vi "LlenarTabla.vi"(8 "error in (no error)":errorcluster, 10 "Tabla":T1(ring), 11 "Prueba32 in":refnum<class "Prueba33.lvclass">) -> (0 "error out":errorcluster, 3 "Prueba32 out":refnum<class "Prueba33.lvclass">)   [LabVIEW 2019, in "Prueba33.lvclass"]
uses:
  Prueba33.lvclass
  Prueba33.lvclass/Prueba33.ctl
panel:
  out "Tabla":string[][](table)=[["63"], ["125"], ["250"], ["500"], ["1000"], ["2000"], ["4000"], ["8000"]]
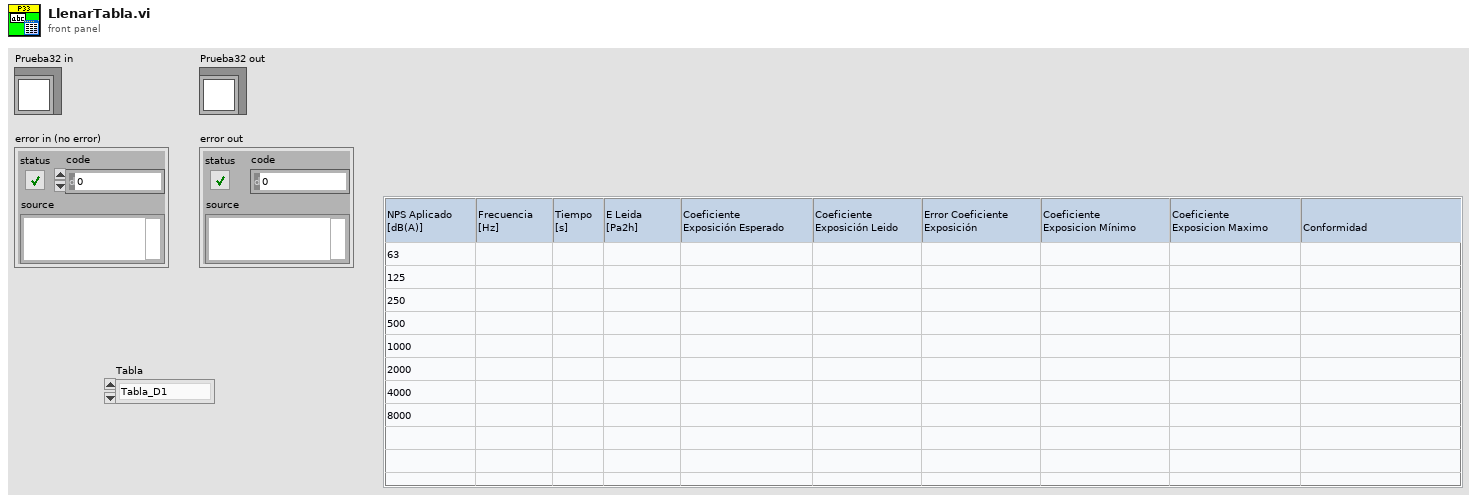
[diagram p1: front panel]
types:
  T1 = enum16{"Tabla_D1", "Tabla_D2", "Tabla_D3", "Tabla_D4"}
  T2 = cluster{"ControlName":string, "ControlReference":refnum<vi>}[]
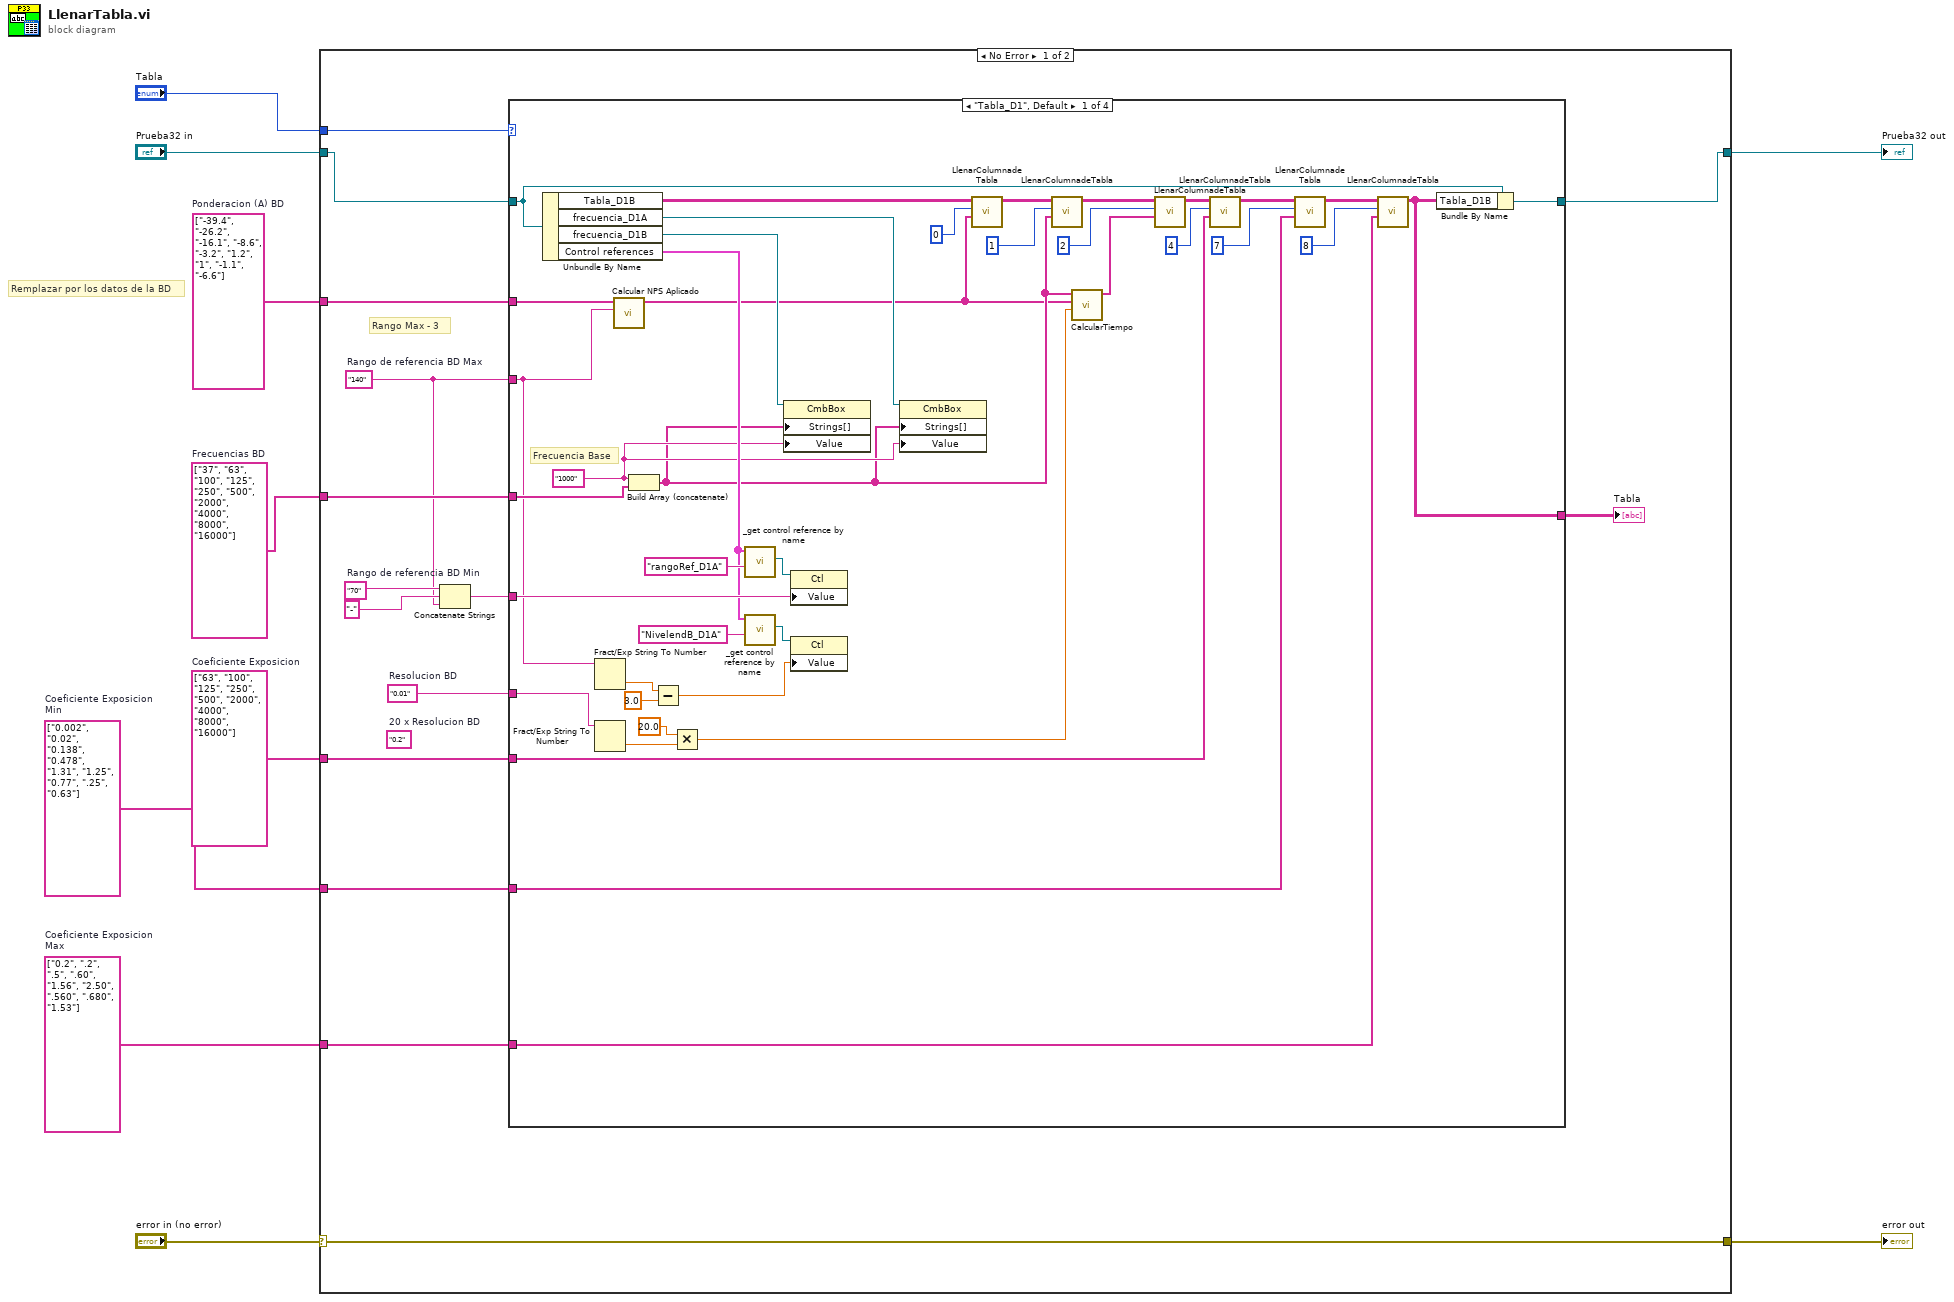
[diagram p0: block diagram]
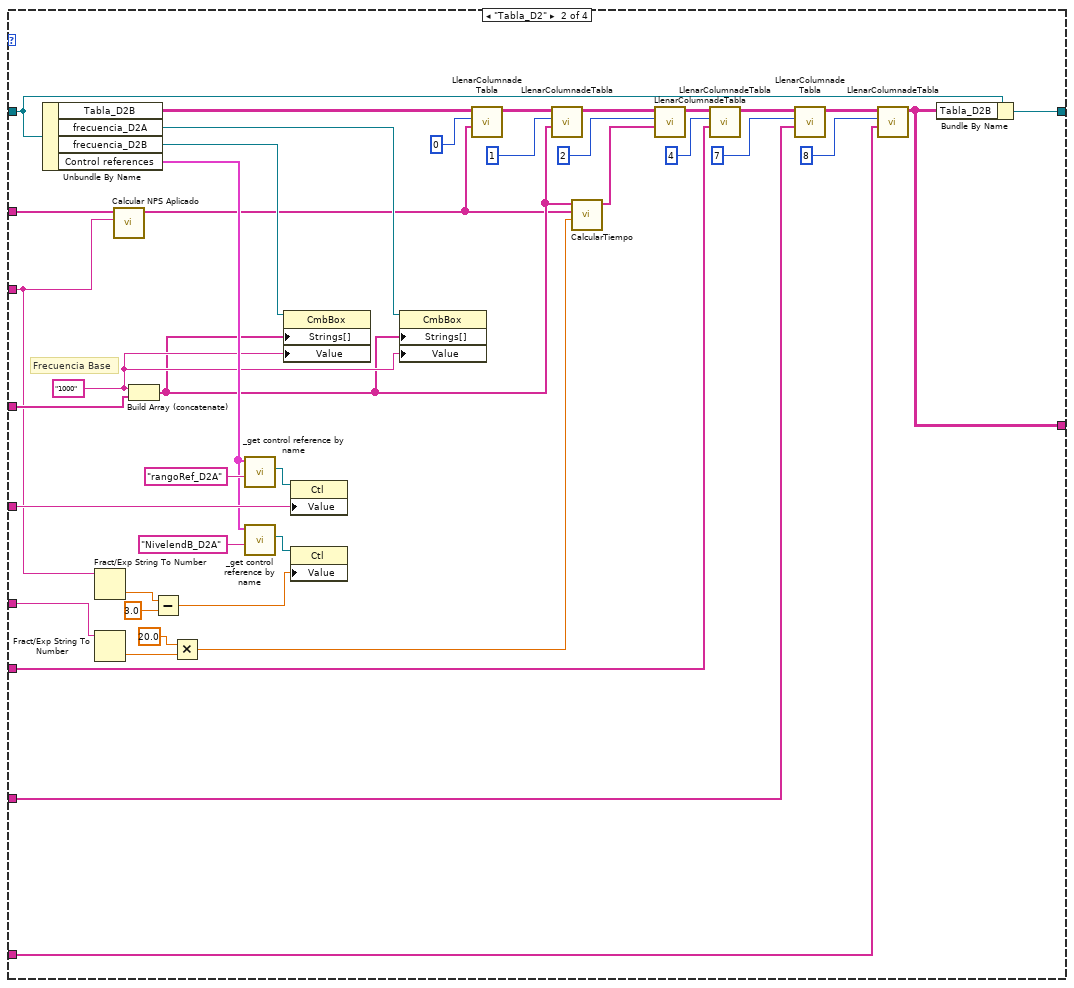
[diagram p2: hidden frame]
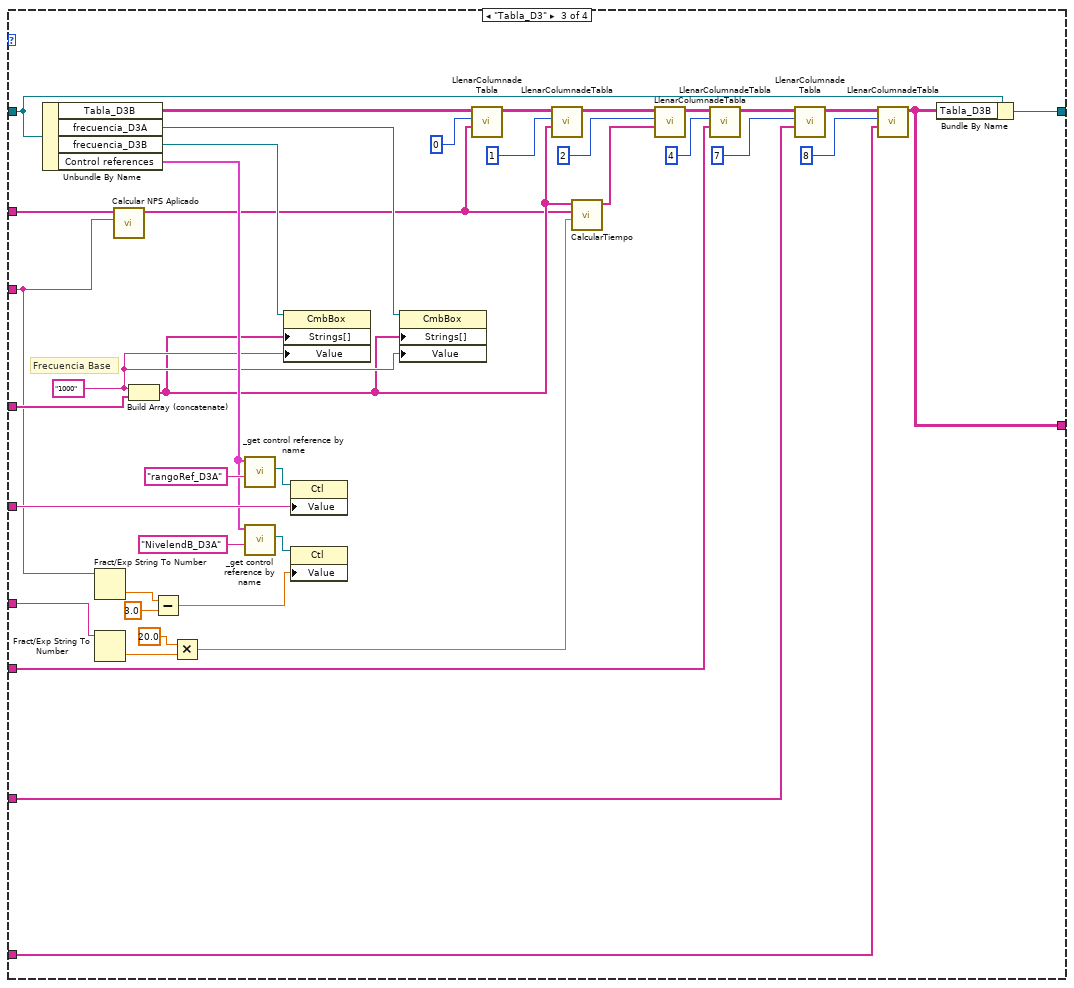
[diagram p3: hidden frame]
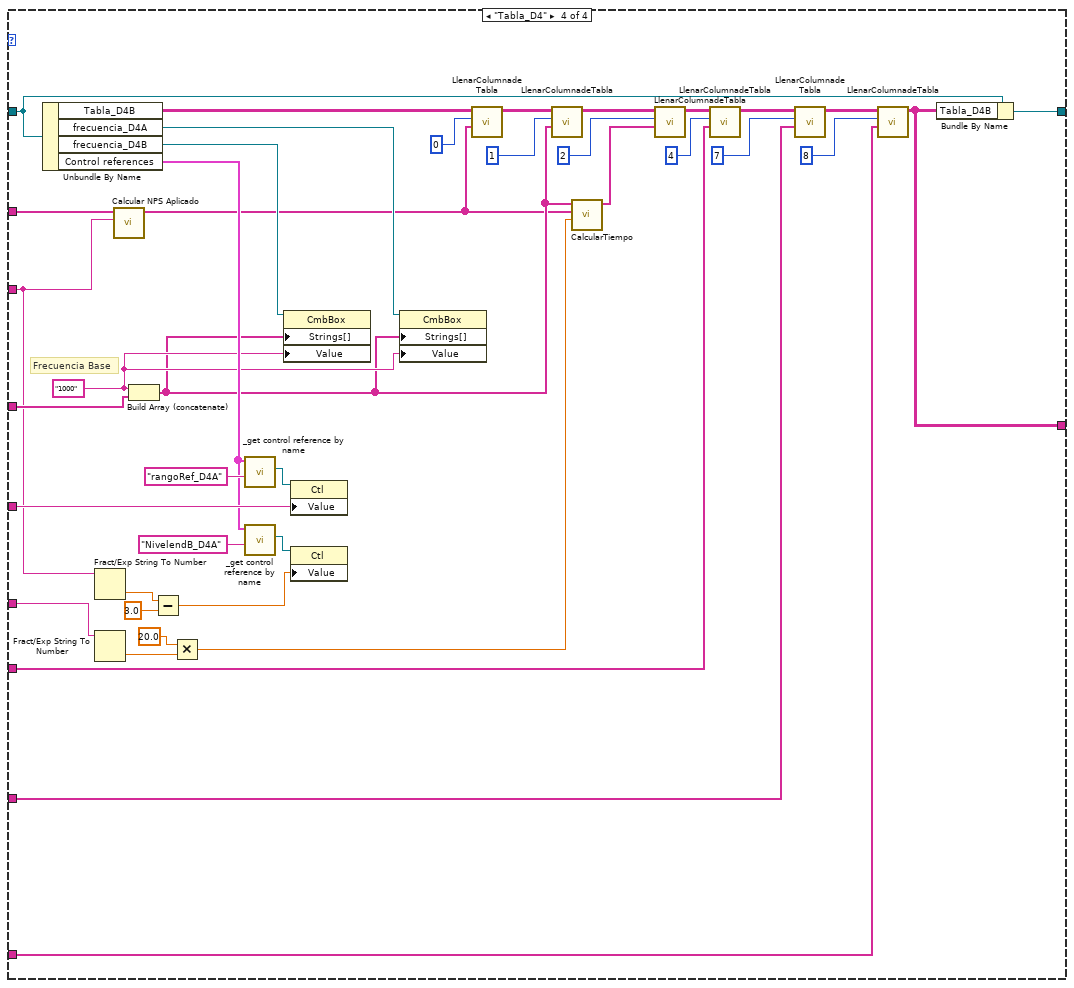
[diagram p4: hidden frame]
diagram:
  w1 = string[] ["0.2", ".2", ".5", ".60", "1.56", "2.50", ".560", ".680", "1.53"]  # Coeficiente Exposicion Max
  w2 = string[] ["0.002", "0.02", "0.138", "0.478", "1.31", "1.25", "0.77", ".25", "0.63"]  # Coeficiente Exposicion Min
  w3 = string[] ["63", "100", "125", "250", "500", "2000", "4000", "8000", "16000"]  # Coeficiente Exposicion
  w4 = string[] ["37", "63", "100", "125", "250", "500", "2000", "4000", "8000", "16000"]  # Frecuencias BD
  w5 = string[] ["-39.4", "-26.2", "-16.1", "-8.6", "-3.2", "1.2", "1", "-1.1", "-6.6"]  # Ponderacion (A) BD
  # "Remplazar por los datos de la BD"
  n1 = case shown="No Error" "error in (no error)" {
    selector: "error in (no error)" -> [w25 w186]
    tunnel: [w25 w186] -> w8
    tunnel: [w24 w187] -> w9
    tunnel: "Prueba32 in" -> [w23 w187]
    tunnel: "Tabla" -> [w22 _]
    tunnel: w5 -> [w21 _]
    tunnel: w4 -> [w20 _]
    tunnel: w3 -> [w19 _]
    tunnel: w2 -> [w18 _]
    tunnel: w1 -> [w17 _]
    frame No Error {
      w11 = "0.01"  # Resolucion BD
      (unwired) "0.2"  # 20 x Resolucion BD
      w12 = "140"  # Rango de referencia BD Max
      w15 = "70"  # Rango de referencia BD Min
      # "Rango Max - 3"
      n2 = Concatenate Strings(w15, "-", w12) -> (w13:string)
      n3 = case shown="\"Tabla_D1\", Default" w22 {
        tunnel: [w64 w104 w144 w184] -> w24
        tunnel: w23 -> [w63 w103 w143 w183]
        tunnel: w12 -> [w40 w80 w120 w160]
        tunnel: w21 -> [w61 w101 w141 w181]
        tunnel: w20 -> [w58 w98 w138 w178]
        tunnel: w19 -> [w54 w94 w134 w174]
        tunnel: w18 -> [w48 w88 w128 w168]
        tunnel: w17 -> [w47 w87 w127 w167]
        tunnel: [w46 w86 w126 w166] -> w16
        tunnel: w13 -> [w43 w83 w123 w163]
        tunnel: w11 -> [w30 w70 w110 w150]
        frame "Tabla_D1", Default {
          w33 = "1000"
          # "Frecuencia Base"
          n4 = Unbundle By Name(w63) -> ("Tabla_D1B"=w65:string[][], "frecuencia_D1A"=w34:refnum<vi>, "frecuencia_D1B"=w35:refnum<vi>, "Control references"=w36:T2)
          n5 = Fract/Exp String To Number(string=w40) -> (number=w39:dbl)  [unwired: 3 in, 1 out]
          n6 = Fract/Exp String To Number(string=w30) -> (number=w29:dbl)  [unwired: 3 in, 1 out]
          n7 = call "Calcular NPS Aplicado.vi"("Rango de MAX de referencia BD"=w40, "Ponderacion BD"=w61) -> ("NPS Aplicado"=w31:string[])  [unwired: 9 in]
          n8 = Build Array (concatenate)(w33, w58) -> (w32:string[])
          n9 = Subtract(x=w39, y=3.0) -> (x-y=w37:dbl)
          n10 = Multiply(x=20.0, y=w29) -> (x*y=w27:dbl)
          n11 = call "_get control reference by name.vi"("Control name"="rangoRef_D1A", "Control references"=w36) -> ("Ctl Refnum"=w44:refnum<vi>)  [unwired: 4 in, 1 out]
          n12 = call "_get control reference by name.vi"("Control name"="NivelendB_D1A", "Control references"=w36) -> ("Ctl Refnum"=w41:refnum<vi>)  [unwired: 4 in, 1 out]
          n13 = property class="CmbBox"(reference=w35, "Strings[]"=w32, "Value"=w33) -> ()  [unwired: 1 in, 2 out]
          n14 = property class="Ctl"(reference=w44, "Value"=w43) -> ()  [unwired: 1 in, 2 out]
          n15 = property class="Ctl"(reference=w41, "Value"=w37) -> ()  [unwired: 1 in, 2 out]
          n16 = property class="CmbBox"(reference=w34, "Strings[]"=w32, "Value"=w33) -> ()  [unwired: 1 in, 2 out]
          n17 = call "LlenarColumnadeTabla.vi"("Data"=w31, "Col. Number"=0, "Tabla in"=w65) -> ("Tabla out"=w59:string[][])  [unwired: 8 in]
          n18 = call "LlenarColumnadeTabla.vi"("Data"=w32, "Col. Number"=1, "Tabla in"=w59) -> ("Tabla out"=w57:string[][])  [unwired: 8 in]
          n19 = call "CalcularTiempo.vi"("20xResolucion"=w27, "NPS Aplicado"=w31, "Frecuencias"=w32) -> ("Tiempo"=w26:string[])  [unwired: 8 in]
          n20 = call "LlenarColumnadeTabla.vi"("Data"=w26, "Col. Number"=2, "Tabla in"=w57) -> ("Tabla out"=w55:string[][])  [unwired: 8 in]
          n21 = call "LlenarColumnadeTabla.vi"("Data"=w54, "Col. Number"=4, "Tabla in"=w55) -> ("Tabla out"=w52:string[][])  [unwired: 8 in]
          n22 = call "LlenarColumnadeTabla.vi"("Data"=w48, "Col. Number"=7, "Tabla in"=w52) -> ("Tabla out"=w51:string[][])  [unwired: 8 in]
          n23 = call "LlenarColumnadeTabla.vi"("Data"=w47, "Col. Number"=8, "Tabla in"=w51) -> ("Tabla out"=w46:string[][])  [unwired: 8 in]
          n24 = Bundle By Name(cluster=w63, "Tabla_D1B"=w46) -> (w64:refnum<class "Prueba33.lvclass">)
        }
        frame "Tabla_D2" {
          w73 = "1000"
          # "Frecuencia Base"
          n25 = Unbundle By Name(w103) -> ("Tabla_D2B"=w105:string[][], "frecuencia_D2A"=w74:refnum<vi>, "frecuencia_D2B"=w75:refnum<vi>, "Control references"=w76:T2)
          n26 = Fract/Exp String To Number(string=w80) -> (number=w79:dbl)  [unwired: 3 in, 1 out]
          n27 = Fract/Exp String To Number(string=w70) -> (number=w69:dbl)  [unwired: 3 in, 1 out]
          n28 = call "Calcular NPS Aplicado.vi"("Rango de MAX de referencia BD"=w80, "Ponderacion BD"=w101) -> ("NPS Aplicado"=w71:string[])  [unwired: 9 in]
          n29 = Build Array (concatenate)(w73, w98) -> (w72:string[])
          n30 = Subtract(x=w79, y=3.0) -> (x-y=w77:dbl)
          n31 = Multiply(x=20.0, y=w69) -> (x*y=w67:dbl)
          n32 = call "_get control reference by name.vi"("Control name"="rangoRef_D2A", "Control references"=w76) -> ("Ctl Refnum"=w84:refnum<vi>)  [unwired: 4 in, 1 out]
          n33 = call "_get control reference by name.vi"("Control name"="NivelendB_D2A", "Control references"=w76) -> ("Ctl Refnum"=w81:refnum<vi>)  [unwired: 4 in, 1 out]
          n34 = property class="CmbBox"(reference=w75, "Strings[]"=w72, "Value"=w73) -> ()  [unwired: 1 in, 2 out]
          n35 = property class="Ctl"(reference=w84, "Value"=w83) -> ()  [unwired: 1 in, 2 out]
          n36 = property class="Ctl"(reference=w81, "Value"=w77) -> ()  [unwired: 1 in, 2 out]
          n37 = property class="CmbBox"(reference=w74, "Strings[]"=w72, "Value"=w73) -> ()  [unwired: 1 in, 2 out]
          n38 = call "LlenarColumnadeTabla.vi"("Data"=w71, "Col. Number"=0, "Tabla in"=w105) -> ("Tabla out"=w99:string[][])  [unwired: 8 in]
          n39 = call "LlenarColumnadeTabla.vi"("Data"=w72, "Col. Number"=1, "Tabla in"=w99) -> ("Tabla out"=w97:string[][])  [unwired: 8 in]
          n40 = call "CalcularTiempo.vi"("20xResolucion"=w67, "NPS Aplicado"=w71, "Frecuencias"=w72) -> ("Tiempo"=w66:string[])  [unwired: 8 in]
          n41 = call "LlenarColumnadeTabla.vi"("Data"=w66, "Col. Number"=2, "Tabla in"=w97) -> ("Tabla out"=w95:string[][])  [unwired: 8 in]
          n42 = call "LlenarColumnadeTabla.vi"("Data"=w94, "Col. Number"=4, "Tabla in"=w95) -> ("Tabla out"=w92:string[][])  [unwired: 8 in]
          n43 = call "LlenarColumnadeTabla.vi"("Data"=w88, "Col. Number"=7, "Tabla in"=w92) -> ("Tabla out"=w91:string[][])  [unwired: 8 in]
          n44 = call "LlenarColumnadeTabla.vi"("Data"=w87, "Col. Number"=8, "Tabla in"=w91) -> ("Tabla out"=w86:string[][])  [unwired: 8 in]
          n45 = Bundle By Name(cluster=w103, "Tabla_D2B"=w86) -> (w104:refnum<class "Prueba33.lvclass">)
        }
        frame "Tabla_D3" {
          w113 = "1000"
          # "Frecuencia Base"
          n46 = Unbundle By Name(w143) -> ("Tabla_D3B"=w145:string[][], "frecuencia_D3A"=w114:refnum<vi>, "frecuencia_D3B"=w115:refnum<vi>, "Control references"=w116:T2)
          n47 = Fract/Exp String To Number(string=w120) -> (number=w119:dbl)  [unwired: 3 in, 1 out]
          n48 = Fract/Exp String To Number(string=w110) -> (number=w109:dbl)  [unwired: 3 in, 1 out]
          n49 = call "Calcular NPS Aplicado.vi"("Rango de MAX de referencia BD"=w120, "Ponderacion BD"=w141) -> ("NPS Aplicado"=w111:string[])  [unwired: 9 in]
          n50 = Build Array (concatenate)(w113, w138) -> (w112:string[])
          n51 = Subtract(x=w119, y=3.0) -> (x-y=w117:dbl)
          n52 = Multiply(x=20.0, y=w109) -> (x*y=w107:dbl)
          n53 = call "_get control reference by name.vi"("Control name"="rangoRef_D3A", "Control references"=w116) -> ("Ctl Refnum"=w124:refnum<vi>)  [unwired: 4 in, 1 out]
          n54 = call "_get control reference by name.vi"("Control name"="NivelendB_D3A", "Control references"=w116) -> ("Ctl Refnum"=w121:refnum<vi>)  [unwired: 4 in, 1 out]
          n55 = property class="CmbBox"(reference=w115, "Strings[]"=w112, "Value"=w113) -> ()  [unwired: 1 in, 2 out]
          n56 = property class="Ctl"(reference=w124, "Value"=w123) -> ()  [unwired: 1 in, 2 out]
          n57 = property class="Ctl"(reference=w121, "Value"=w117) -> ()  [unwired: 1 in, 2 out]
          n58 = property class="CmbBox"(reference=w114, "Strings[]"=w112, "Value"=w113) -> ()  [unwired: 1 in, 2 out]
          n59 = call "LlenarColumnadeTabla.vi"("Data"=w111, "Col. Number"=0, "Tabla in"=w145) -> ("Tabla out"=w139:string[][])  [unwired: 8 in]
          n60 = call "LlenarColumnadeTabla.vi"("Data"=w112, "Col. Number"=1, "Tabla in"=w139) -> ("Tabla out"=w137:string[][])  [unwired: 8 in]
          n61 = call "CalcularTiempo.vi"("20xResolucion"=w107, "NPS Aplicado"=w111, "Frecuencias"=w112) -> ("Tiempo"=w106:string[])  [unwired: 8 in]
          n62 = call "LlenarColumnadeTabla.vi"("Data"=w106, "Col. Number"=2, "Tabla in"=w137) -> ("Tabla out"=w135:string[][])  [unwired: 8 in]
          n63 = call "LlenarColumnadeTabla.vi"("Data"=w134, "Col. Number"=4, "Tabla in"=w135) -> ("Tabla out"=w132:string[][])  [unwired: 8 in]
          n64 = call "LlenarColumnadeTabla.vi"("Data"=w128, "Col. Number"=7, "Tabla in"=w132) -> ("Tabla out"=w131:string[][])  [unwired: 8 in]
          n65 = call "LlenarColumnadeTabla.vi"("Data"=w127, "Col. Number"=8, "Tabla in"=w131) -> ("Tabla out"=w126:string[][])  [unwired: 8 in]
          n66 = Bundle By Name(cluster=w143, "Tabla_D3B"=w126) -> (w144:refnum<class "Prueba33.lvclass">)
        }
        frame "Tabla_D4" {
          w153 = "1000"
          # "Frecuencia Base"
          n67 = Unbundle By Name(w183) -> ("Tabla_D4B"=w185:string[][], "frecuencia_D4A"=w154:refnum<vi>, "frecuencia_D4B"=w155:refnum<vi>, "Control references"=w156:T2)
          n68 = Fract/Exp String To Number(string=w160) -> (number=w159:dbl)  [unwired: 3 in, 1 out]
          n69 = Fract/Exp String To Number(string=w150) -> (number=w149:dbl)  [unwired: 3 in, 1 out]
          n70 = call "Calcular NPS Aplicado.vi"("Rango de MAX de referencia BD"=w160, "Ponderacion BD"=w181) -> ("NPS Aplicado"=w151:string[])  [unwired: 9 in]
          n71 = Build Array (concatenate)(w153, w178) -> (w152:string[])
          n72 = Subtract(x=w159, y=3.0) -> (x-y=w157:dbl)
          n73 = Multiply(x=20.0, y=w149) -> (x*y=w147:dbl)
          n74 = call "_get control reference by name.vi"("Control name"="rangoRef_D4A", "Control references"=w156) -> ("Ctl Refnum"=w164:refnum<vi>)  [unwired: 4 in, 1 out]
          n75 = call "_get control reference by name.vi"("Control name"="NivelendB_D4A", "Control references"=w156) -> ("Ctl Refnum"=w161:refnum<vi>)  [unwired: 4 in, 1 out]
          n76 = property class="CmbBox"(reference=w155, "Strings[]"=w152, "Value"=w153) -> ()  [unwired: 1 in, 2 out]
          n77 = property class="Ctl"(reference=w164, "Value"=w163) -> ()  [unwired: 1 in, 2 out]
          n78 = property class="Ctl"(reference=w161, "Value"=w157) -> ()  [unwired: 1 in, 2 out]
          n79 = property class="CmbBox"(reference=w154, "Strings[]"=w152, "Value"=w153) -> ()  [unwired: 1 in, 2 out]
          n80 = call "LlenarColumnadeTabla.vi"("Data"=w151, "Col. Number"=0, "Tabla in"=w185) -> ("Tabla out"=w179:string[][])  [unwired: 8 in]
          n81 = call "LlenarColumnadeTabla.vi"("Data"=w152, "Col. Number"=1, "Tabla in"=w179) -> ("Tabla out"=w177:string[][])  [unwired: 8 in]
          n82 = call "CalcularTiempo.vi"("20xResolucion"=w147, "NPS Aplicado"=w151, "Frecuencias"=w152) -> ("Tiempo"=w146:string[])  [unwired: 8 in]
          n83 = call "LlenarColumnadeTabla.vi"("Data"=w146, "Col. Number"=2, "Tabla in"=w177) -> ("Tabla out"=w175:string[][])  [unwired: 8 in]
          n84 = call "LlenarColumnadeTabla.vi"("Data"=w174, "Col. Number"=4, "Tabla in"=w175) -> ("Tabla out"=w172:string[][])  [unwired: 8 in]
          n85 = call "LlenarColumnadeTabla.vi"("Data"=w168, "Col. Number"=7, "Tabla in"=w172) -> ("Tabla out"=w171:string[][])  [unwired: 8 in]
          n86 = call "LlenarColumnadeTabla.vi"("Data"=w167, "Col. Number"=8, "Tabla in"=w171) -> ("Tabla out"=w166:string[][])  [unwired: 8 in]
          n87 = Bundle By Name(cluster=w183, "Tabla_D4B"=w166) -> (w184:refnum<class "Prueba33.lvclass">)
        }
      }
      "Tabla" <- w16
    }
    frame Error {
    }
  }
  "Prueba32 out" <- w9
  "error out" <- w8
